vi "Shift Display.vi"(6 "chip select  (1st chip)":enum16{"1st chip", "2nd chip"}(ring), 8 "error in (no error)":errorcluster, 10 "direction":enum16{"left", "right"}(ring), 11 "LCD in":refnum<class "Character LCD.lvclass">) -> (0 "error out":errorcluster, 3 "LCD out":refnum<class "Character LCD.lvclass">)   [LabVIEW 2015, in "HD44780 Host.lvlib"]
uses:
  HD44780 Host.lvlib
  Internal/LCD Class/Character LCD.lvclass
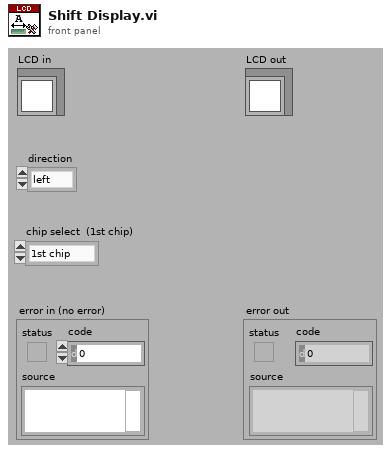
[diagram p1: front panel]
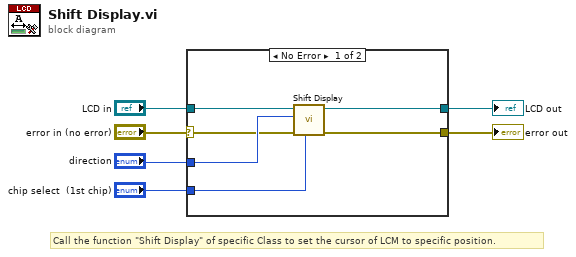
[diagram p0: block diagram]
diagram:
  # "Call the function \"Shift Display\" of specific Class to set the cursor of LCM to specific position."
  n1 = case shown="No Error" "error in (no error)" {
    selector: "error in (no error)" -> [w7 w14]
    tunnel: "direction" -> [w12 _]
    tunnel: "chip select  (1st chip)" -> [w11 _]
    tunnel: [w8 w14] -> w4
    tunnel: "LCD in" -> [w10 w13]
    tunnel: [w9 w13] -> w1
    frame No Error {
      n2 = call-dynamic "Shift Display.vi"("chip select  (1st chip)"=w11, "error in (no error)"=w7, "direction"=w12, "Character LCD in"=w10) -> ("error out"=w8:errorcluster, "Character LCD out"=w9:refnum<class "Character LCD.lvclass">)  [unwired: 6 in]
    }
    frame Error {
    }
  }
  "error out" <- w4
  "LCD out" <- w1
